vi "RoboMirror.vi"(6 "threads (8)":u8=8, 8 "error in":errorcluster, 9 "Log Path":path, 10 "Dest Path":path, 11 "Source Path":path) -> (0 "error out":errorcluster)   [LabVIEW 2023]
panel:
  out "file in tmp dir":path
  out "standard error":string
  out "standard output":string
  out "String":string
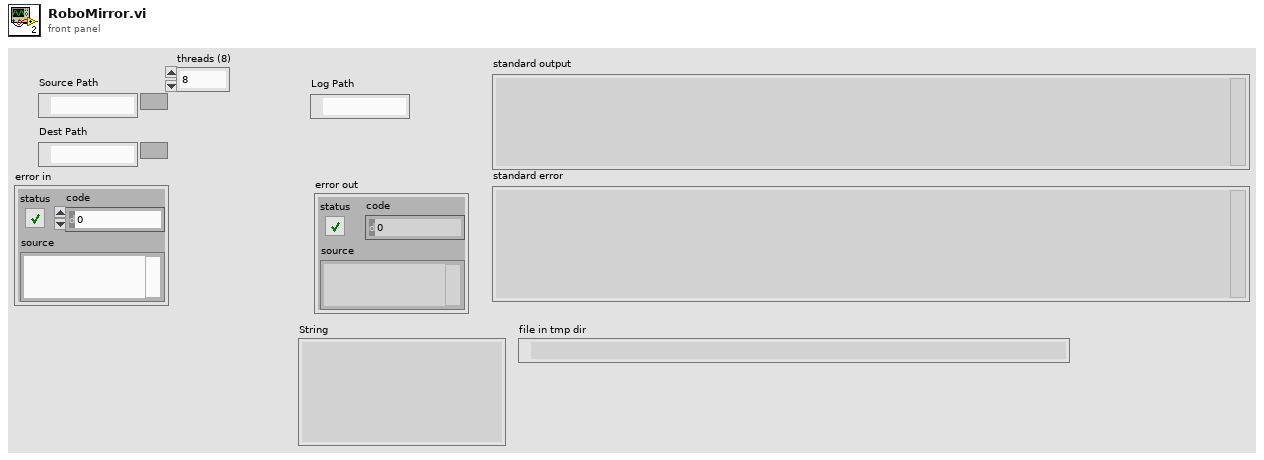
[diagram p1: front panel]
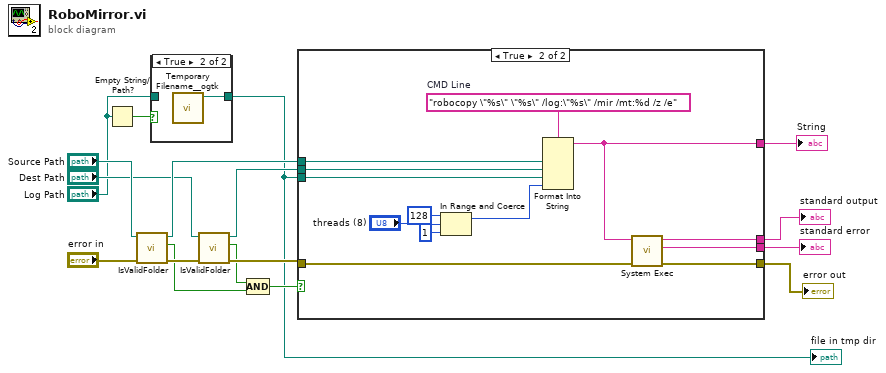
[diagram p0: block diagram]
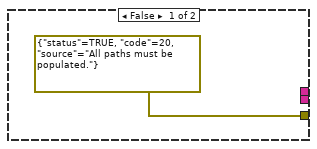
[diagram p3: hidden frame]
diagram:
  n1 = Empty String/Path?(string/path="Log Path") -> (empty?=w5:bool)
  n2 = call "IsValidFolder.vi"("error in (no error)"="error in", "Source Path"="Source Path") -> ("error out"=w12:errorcluster, "Valid Folder"=w9:bool, "path out"=w15:path)  [unwired: 7 in]
  n3 = case shown="True" w5 {
    tunnel: [w18 w19] -> w4
    tunnel: "Log Path" -> [w18 _]
    frame False {
    }
    frame True {
      n4 = call <userlib>:"Temporary Filename__ogtk.vi"() -> ("file in tmp dir"=w19:path)  [unwired: 6 in, 1 out]
    }
  }
  "file in tmp dir" <- w4
  n5 = call "IsValidFolder.vi"("error in (no error)"=w12, "Source Path"="Dest Path") -> ("error out"=w11:errorcluster, "Valid Folder"=w10:bool, "path out"=w13:path)  [unwired: 7 in]
  n6 = Compound Arithmetic op=AND(w10, w9) -> (w8:bool)
  n7 = case shown="True" w8 {
    tunnel: w15 -> [_ w28]
    tunnel: w13 -> [_ w27]
    tunnel: w4 -> [_ w26]
    tunnel: [errorcluster {"status"=TRUE, "code"=20, "source"="All paths must be populated."} ("error out") w24] -> w7
    tunnel: w11 -> [_ w25]
    tunnel: [_ w23] -> w6
    tunnel: [_ w22] -> w2
    tunnel: [_ w21] -> w1
    frame False {
    }
    frame True {
      w33 = "robocopy \"%s\" \"%s\" /log:\"%s\" /mir /mt:%d /z /e"  # CMD Line
      n8 = In Range and Coerce(upper limit=u8 128, x="threads (8)", lower limit=u8 1) -> (coerced(x)=w29:u8)  [unwired: 1 out]
      n9 = Format Into String(format string=w33, w28, w27, w26, w29) -> (resulting string=w23:string)  [unwired: 2 in, 1 out]
      n10 = call <vilib>:"System Exec.vi"("error in (no error)"=w25, "command line"=w23) -> ("error out"=w24:errorcluster, "standard error"=w21:string, "standard output"=w22:string)  [unwired: 6 in, 1 out]
    }
  }
  "error out" <- w7
  "String" <- w6
  "standard output" <- w2
  "standard error" <- w1
